vi "WLAN TxP Config.vi"(0 "Instrument Handle In":refnum<k21>, 1 "Selector String":string, 5 "WLAN TxP Config":T1={"Averaging Enabled"=0, "Averaging Count"=10, "Maximum Measurement Interval (s)"=0.0} {"Maximum Measurement Interval (s)" format="%.3p"; "Averaging Enabled" items=["False", "True"]}, 11 "error in (no error)":errorcluster) -> (4 "Instrument Handle Out":refnum<k21>, 15 "error out":errorcluster)   [LabVIEW 2018, in "RFmxWLAN.lvlib"]
uses:
  RFmxWLAN.lvlib
  Typedefs/WLAN TxP Config.ctl
  <resource>/objmgr/RFmxWLAN.rc
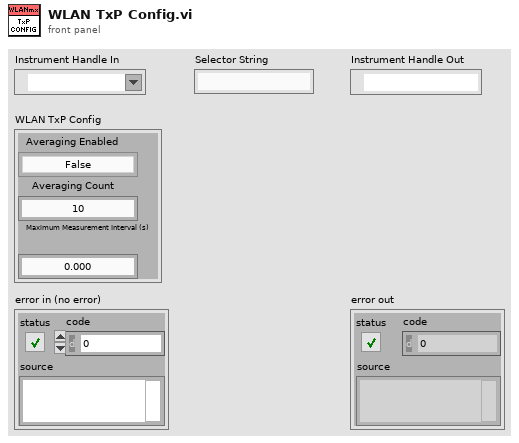
[diagram p1: front panel]
types:
  T1 = typedef "RFmxWLAN.lvlib/WLAN TxP Config.ctl" = cluster{"Averaging Enabled":i32, "Averaging Count":i32, "Maximum Measurement Interval (s)":dbl}
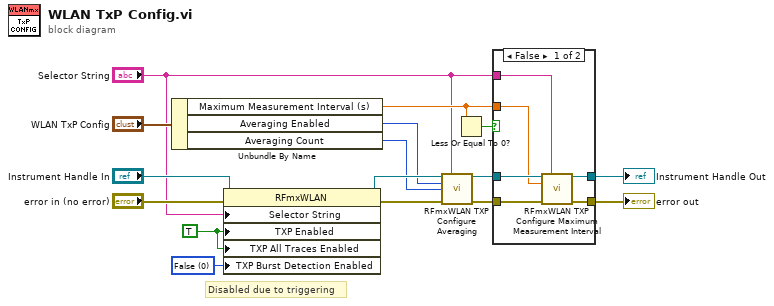
[diagram p0: block diagram]
diagram:
  w1 = 0 items=["False", "True"] ("TXP Burst Detection Enabled")
  w3 = TRUE ("TXP Enabled")
  # "Disabled due to triggering"
  n1 = Unbundle By Name("WLAN TxP Config") -> ("Maximum Measurement Interval (s)"=w4:dbl, "Averaging Enabled"=w6:i32, "Averaging Count"=w5:i32)
  n2 = property class="RFmxWLAN"(reference="Instrument Handle In", error in="error in (no error)", "Selector String"="Selector String", "TXP Enabled"=w3, "TXP All Traces Enabled"=w3, "TXP Burst Detection Enabled"=w1) -> (reference out=w8:refnum<k21>, error out=w13:errorcluster)
  n3 = call <vilib>:"RFmxWLAN TXP Configure Averaging.vi"("Instrument Handle In"=w8, "Selector String"="Selector String", "Averaging Enabled"=w6, "Averaging Count"=w5, "error in (no error)"=w13) -> ("Instrument Handle Out"=w9:refnum<k21>, "error out"=w10:errorcluster)  [unwired: 9 in]
  n4 = Less Or Equal To 0?(x=w4) -> (x <= 0?=w14:bool)
  n5 = case shown="False" w14 {
    tunnel: [w19 w24] -> w12
    tunnel: w9 -> [w20 w24]
    tunnel: [w21 w23] -> w11
    tunnel: w10 -> [w22 w23]
    tunnel: "Selector String" -> [w18 _]
    tunnel: w4 -> [w17 _]
    frame False {
      n6 = call <vilib>:"RFmxWLAN TXP Configure Maximum Measurement Interval.vi"("Instrument Handle In"=w20, "Selector String"=w18, "Maximum Measurement Interval (s)"=w17, "error in (no error)"=w22) -> ("Instrument Handle Out"=w19:refnum<k21>, "error out"=w21:errorcluster)  [unwired: 10 in]
    }
    frame True {
    }
  }
  "Instrument Handle Out" <- w12
  "error out" <- w11
